vi "test Receive Message Abort.vi"(8 "error in (no error)":errorcluster, 11 "TestCase in":refnum<class "Test Network Stream Transmission.lvclass">) -> (0 "error out":errorcluster, 3 "TestCase out":refnum<class "Test Network Stream Transmission.lvclass">)   [LabVIEW 2020, in "Test Network Stream Transmission.lvclass"]
uses:
  Test Network Stream Transmission.lvclass
  <vilib>/addons/_JKI Toolkits/VI Tester/TestCase.llb/TestCase.lvclass
  Source/Protocols/Network Stream Strategy/Network Stream Initiator/Network Stream Initiator.lvclass
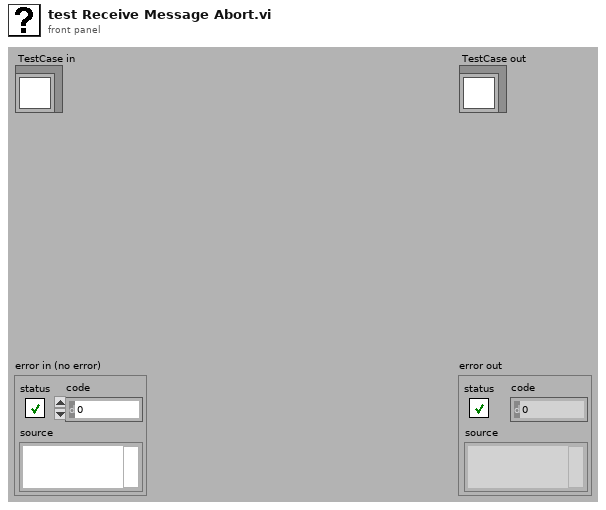
[diagram p1: front panel]
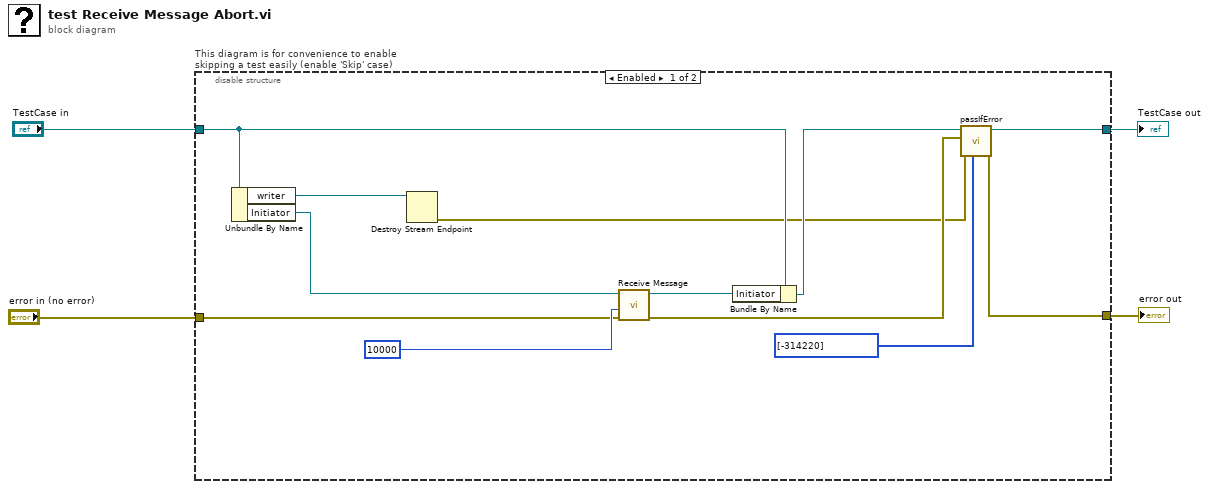
[diagram p0: block diagram]
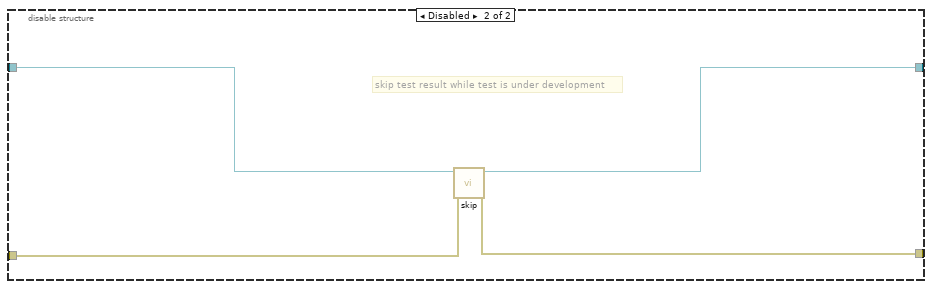
[diagram p2: hidden frame]
diagram:
  n1 = disable-structure "This diagram is for convenience to enable skipping a test easily (enable 'Skip' case)" shown="Enabled" {
    disable-tunnel: "TestCase in" -> [w16 w20]
    disable-tunnel: [w13 w18] -> w1
    disable-tunnel: [w10 w19] -> w3
    disable-tunnel: "error in (no error)" -> [w8 w17]
    frame Enabled {
      n2 = Unbundle By Name(w16) -> ("writer"=w6:refnum<k21>, "Initiator"=w7:refnum<class "Network Stream Initiator.lvclass">)
      n3 = Destroy Stream Endpoint(11:w6) -> (0:w5:errorcluster)  [unwired: 1 in]
      n4 = call-dynamic "Receive Message.vi"("error in (no error)"=w8, "timeout ms (-1)"=10000, "Network Stream in"=w7) -> ("error out"=w11:errorcluster, "Network Stream out"=w14:refnum<class "Network Stream Initiator.lvclass">)  [unwired: 4 in, 3 out]
      n5 = Bundle By Name(cluster=w16, "Initiator"=w14) -> (w15:refnum<class "Test Network Stream Transmission.lvclass">)
      n6 = call-dynamic "passIfError.vi"("passing error codes (default = any error code)"=i32[] [-314220], "error in (no error)"=w5, "error"=w11, "TestCase in"=w15) -> ("error out"=w10:errorcluster, "TestCase out"=w13:refnum<class "Test Network Stream Transmission.lvclass">)  [unwired: 6 in]
    }
    frame Disabled {
      # "skip test result while test is under development"
      n7 = call <vilib>:"skip.vi"("error in (no error)"=w17, "TestCase in"=w20) -> ("error out"=w19:errorcluster, "TestCase out"=w18:refnum<class "Test Network Stream Transmission.lvclass">)  [unwired: 8 in]
    }
  }
  "error out" <- w3
  "TestCase out" <- w1
